vi "Get Read Out Time.vi"(11 "ReadOutTime":sgl) -> (2 "function return":u32, 3 "ReadOutTime out":sgl)   [LabVIEW 2018, in "Copy of Andor SDK.lvlib"]
doc: "EXPNETTYPE unsigned int WINAPI GetReadOutTime(float * ReadOutTime);"
uses:
  Copy of Andor SDK.lvlib
  <userlib>/Andor SDK/ATMCD32D.dll
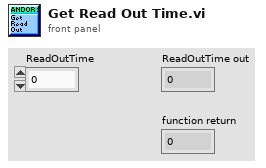
[diagram p1: front panel]
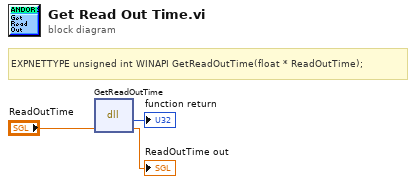
[diagram p0: block diagram]
diagram:
  # "EXPNETTYPE unsigned int WINAPI GetReadOutTime(float * ReadOutTime);"
  n1 = dll-call lib="C:/Program Files (x86)/National Instruments/LabVIEW 2018/user.lib/Andor SDK/ATMCD32D.*" fn="GetReadOutTime"("ReadOutTime"="ReadOutTime") -> (→"function return":u32, "ReadOutTime"=→"ReadOutTime out":sgl)  [unwired: 3 in, 2 out]
